vi "SQL穿管型号数据库读取.vi"(8 "error in (no error)":errorcluster caption="错误输入（无错误）") -> (0 "error out":errorcluster caption="错误输出", 1 "已删除的部分":string[](array[string]), 2 "Type_c":string, 3 "x > 0?":bool, 4 "元素":string)   [LabVIEW 2017]
panel:
  out "Data":string[][](array[string])
  out "子数组":string[](array[string])
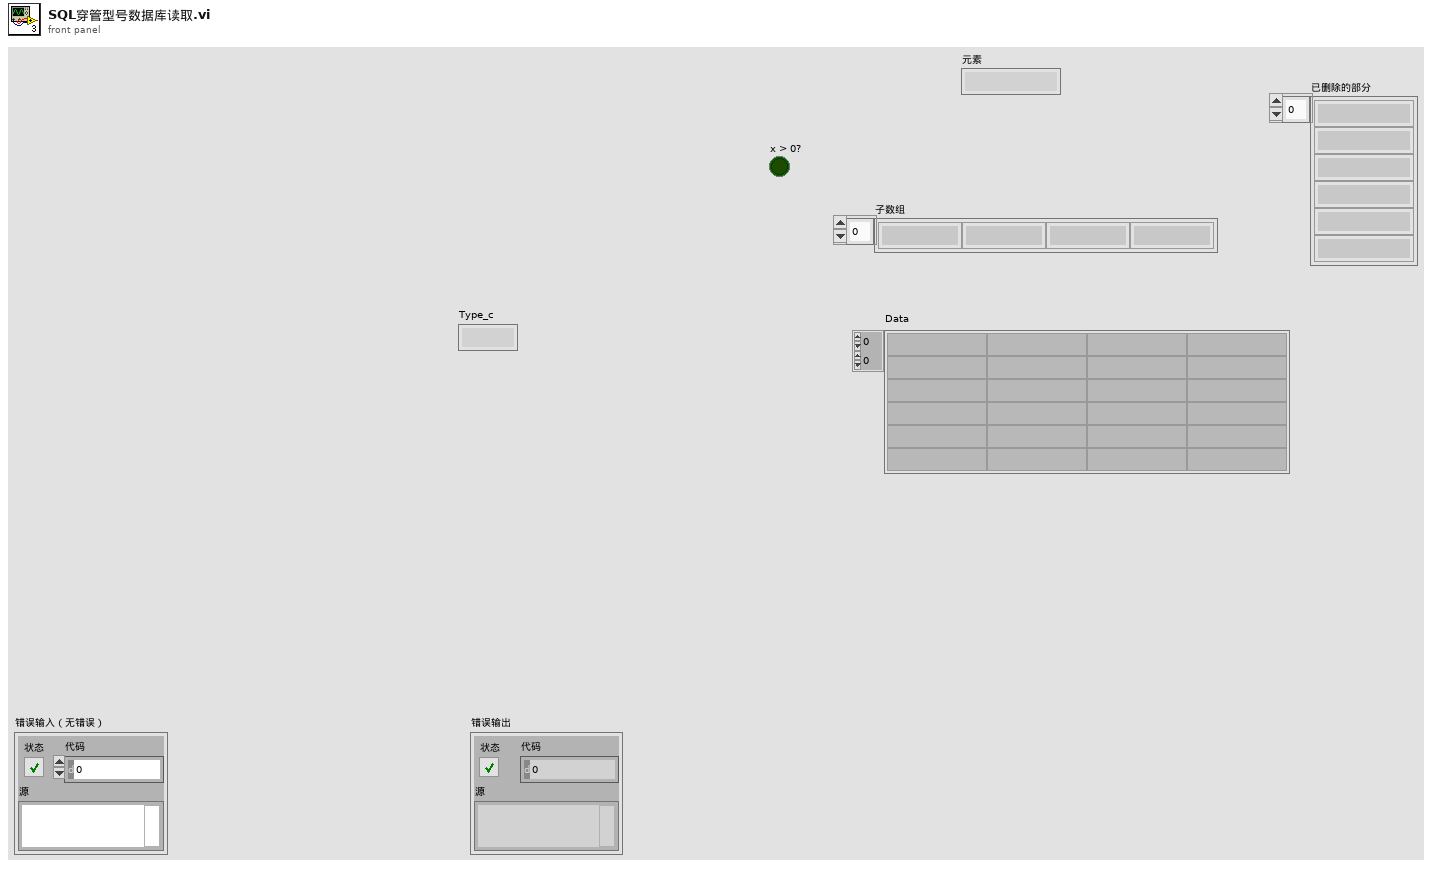
[diagram p1: front panel]
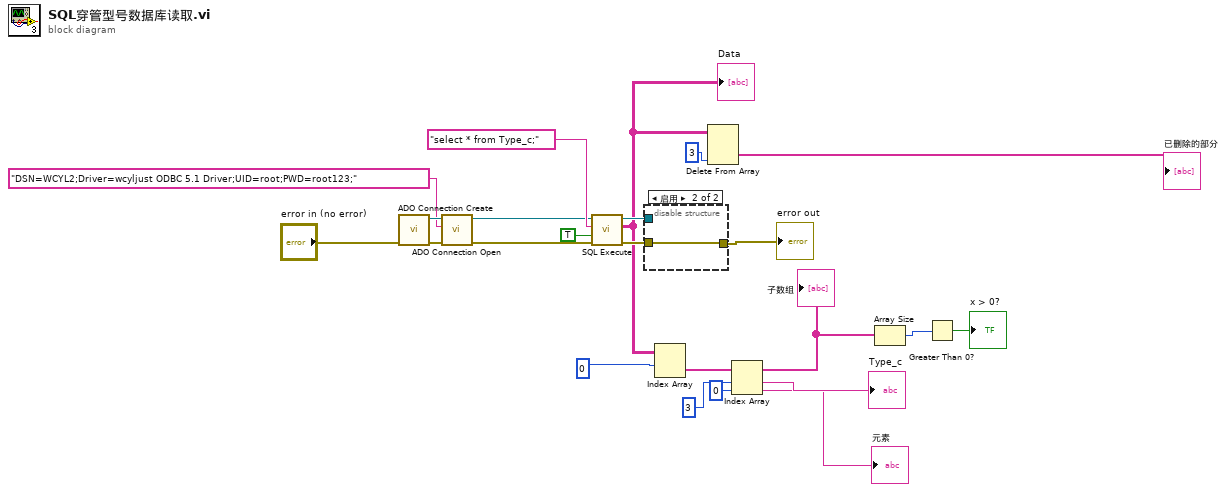
[diagram p0: block diagram]
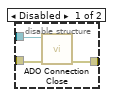
[diagram p2: hidden frame]
diagram:
  n1 = call <userlib>:"ADO Connection Create.vi"("error in (no error)"="error in (no error)") -> ("error out"=w21:errorcluster, "ADODB._Connection Out"=w22:refnum<k7>)  [unwired: 9 in]
  n2 = call <userlib>:"ADO Connection Open.vi"("error in (no error)"=w21, "ConnectionString"="DSN=WCYL2;Driver=wcyljust ODBC 5.1 Driver;UID=root;PWD=root123;", "ADODB._Connection In"=w22) -> ("error out"=w13:errorcluster, "ADODB._Connection Out"=w14:refnum<k7>)  [unwired: 7 in]
  n3 = call <userlib>:"SQL Execute.vi"("error in (no error)"=w13, "Return Data (T)"=TRUE, "Command Text"="select * from Type_c;", "ADODB._Connection In"=w14) -> ("error out"=w11:errorcluster, "Data"=w5:string[][], "ADODB._Connection Out"=w12:refnum<k7>)  [unwired: 4 in, 1 out]
  "Data" <- w5
  n4 = disable-structure shown="启用" {
    disable-tunnel: [w25 w26] -> w18
    disable-tunnel: w12 -> [w24 _]
    disable-tunnel: w11 -> [w23 w26]
    frame Disabled {
      n5 = call <userlib>:"ADO Connection Close.vi"("error in (no error)"=w23, "ADODB._Connection In"=w24) -> ("error out"=w25:errorcluster)  [unwired: 8 in, 1 out]
    }
    frame Enabled {
    }
  }
  "error out" <- w18
  n6 = Index Array(array=w5, index (row)=0 ("索引 (行)")) -> (element=w9:string[])  [unwired: 1 in]
  "子数组" <- w9
  n7 = Delete From Array(array=w5, index (col)=3 ("索引 (行)")) -> (deleted portion=→"已删除的部分":string[])  [unwired: 2 in, 1 out]
  n8 = Index Array(array=w9, index #1=3 ("索引"), index #2=0 ("索引")) -> (element #1=→"Type_c":string, element #2=→"元素":string)
  n9 = Array Size(array=w9) -> (size(s)=w8:i32)
  n10 = Greater Than 0?(x=w8) -> (x > 0?=→"x > 0?":bool)
